vi "Get Current UAV GPS.vi"(8 "Error In":errorcluster) -> (0 "Error Out":errorcluster, 2 "Longitude (degrees)":dbl, 3 "Latitude (degrees)":dbl)   [LabVIEW 2014]
uses:
  Selected Aircraft/SubVI/Get Selected Aircraft.vi
  Get Aircraft Information.vi
  Get Aircraft GPS.vi
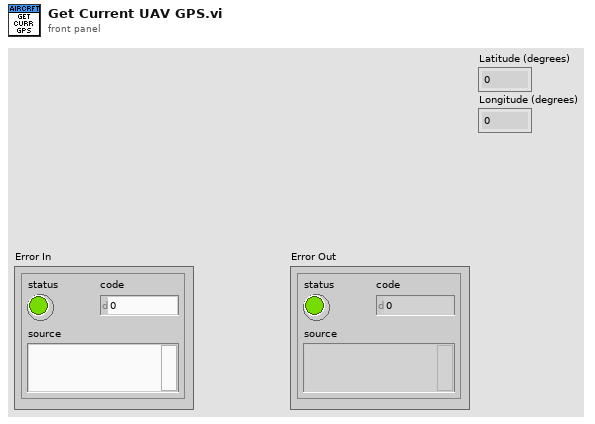
[diagram p1: front panel]
types:
  T1 = typedef "Drone Information.ctl" = cluster{"Aircraft ID":u8, "Tag ID":string, "System Status":string, "Base Mode":T2, "Armed/Disarmed":bool, "Battery Voltage":dbl, "Control Mode":T3, "Initialisation":u8, "Coms with aircraft good":bool, "Mode":string, "Mission Uploaded":bool}
  T2 = typedef "Base Mode.ctl" = cluster{"Custom Mode":bool, "Test Enabled":bool, "Autonomous Mode":bool, "Guided Mode":bool, "Stabilization Enabled":bool, "HIL Enabled":bool, "Manual Mode":bool, "Arm":bool}
  T3 = typedef "Aircraft Mode.ctl" = enum16{"Loiter", "Stabalise", "Failsafe", "Emergency Stop"}
  T4 = typedef "Aircraft GPS Data.ctl" = cluster{"Latitude (degrees)":dbl, "Longitude (degrees)":dbl, "Altitude (m)":dbl, "Fix Type":T5, "HDOP (cm)":u16, "VDOP (cm)":u16, "Ground Speed (m/s)":dbl, "Coarse Over Ground (degrees)":u16, "Number of Satellites":u8}
  T5 = typedef "GPS Fix Type.ctl" = enum16{"No Fix 0", "No Fix 1", "2D Fix", "3D Fix", "DGPS", "RTK"}
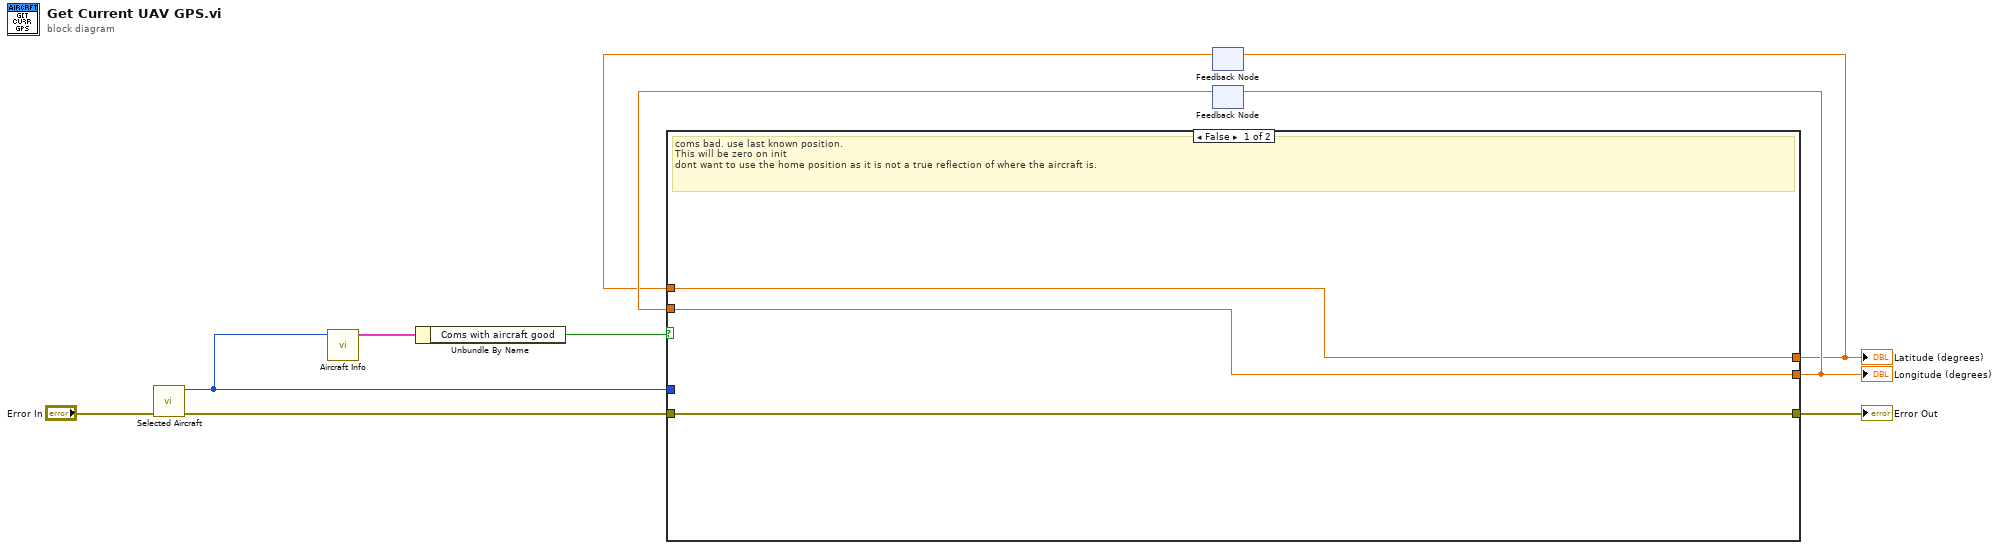
[diagram p0: block diagram]
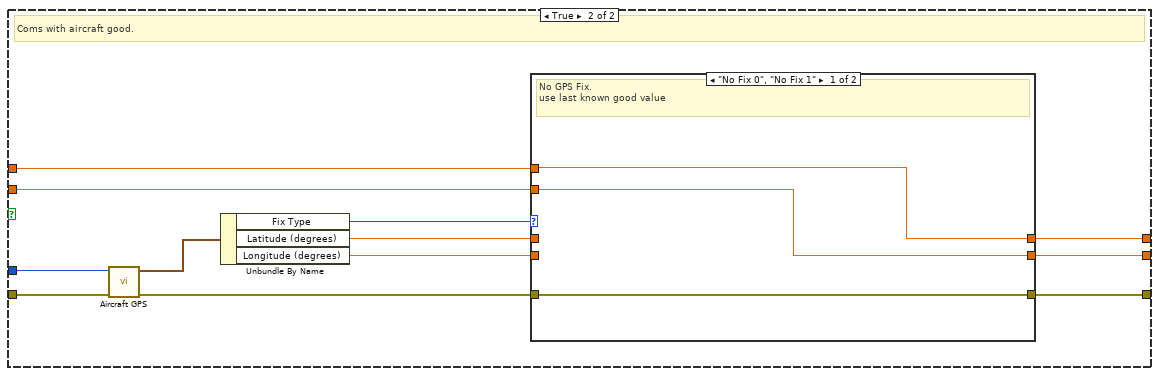
[diagram p2: hidden frame]
diagram:
  n1 = call-poly "Selected Aircraft.vi"("Error In"="Error In") -> ("Error Out"=w9:errorcluster, "Selected Aircraft ID Out"=w6:u8)  [unwired: 9 in]
  n2 = call-poly "Aircraft Info.vi"("Aircraft ID"=w6) -> ("Aircraft Information Out"=w8:T1)  [unwired: 9 in, 1 out]
  n3 = Unbundle By Name(w8) -> ("Coms with aircraft good"=w5:bool)
  n4 = feedback #1() -> (w1:dbl)  [unwired: 1 in]
  n5 = feedback #2() -> (w2:dbl)  [unwired: 1 in]
  n6 = case shown="False" w5 {
    tunnel: w9 -> [w13 w24]
    tunnel: [w12 w20] -> w3
    tunnel: [w11 w19] -> w4
    tunnel: [w13 w18] -> w7
    tunnel: w6 -> [_ w17]
    tunnel: w2 -> [w11 w14]
    tunnel: w1 -> [w12 w15]
    frame False {
      # "coms bad. use last known position. \nThis will be zero on init\ndont want to use the home position as it is not a true reflection of where the aircraft is."
    }
    frame True {
      # "Coms with aircraft good."
      n7 = call-poly "Aircraft GPS.vi"("Error In"=w24, "Aircraft ID"=w17) -> ("Error Out"=w23:errorcluster, "Aircraft GPS Data Out"=w25:T4)  [unwired: 8 in]
      n8 = Unbundle By Name(w25) -> ("Fix Type"=w16:T5, "Latitude (degrees)"=w22:dbl, "Longitude (degrees)"=w21:dbl)
      n9 = case shown="\"No Fix 0\", \"No Fix 1\"" w16 {
        tunnel: w23 -> [w26 w29]
        tunnel: w22 -> [_ w31]
        tunnel: w21 -> [_ w30]
        tunnel: [w28 w31] -> w20
        tunnel: [w27 w30] -> w19
        tunnel: [w26 w29] -> w18
        tunnel: w15 -> [w28 _]
        tunnel: w14 -> [w27 _]
        frame "No Fix 0", "No Fix 1" {
          # "No GPS Fix.\nuse last known good value"
        }
        frame "2D Fix", Default {
          # "Anything other than no fix"
        }
      }
    }
  }
  "Error Out" <- w7
  "Latitude (degrees)" <- w3
  "Longitude (degrees)" <- w4
  n10 = feedback-in #1(w3) -> ()
  n11 = feedback-in #2(w4) -> ()
